vi "Draw Functions.vi"() -> ()   [LabVIEW 2018]
doc: "Draw Functions: This example is an example of drawing functions, demonstrating how to draw lines, rectangles, ellipses, circles, etc."
uses:
  vi.lib/VIRobotics/opencv_yiku/ctls/Size.ctl
  vi.lib/VIRobotics/opencv_yiku/Mat/Create_Mat_8UC3_Size.vi
  vi.lib/VIRobotics/opencv_yiku/opencv_yiku.lvlib
panel:
  in  "pts":cluster{"x":i32, "y":i32}[](array[cluster])
  in  "text":string
  in  "text point":cluster{"x":i32, "y":i32}
  in  "ellipse axes":T1
  in  "ellipse center":cluster{"x":i32, "y":i32}
  in  "circle radius":i32=1
  in  "circle center":cluster{"x":i32, "y":i32}={"x"=200, "y"=200}
  in  "end pt2":cluster{"x":i32, "y":i32}={"x"=350, "y"=270}
  in  "rect":T2={"x"=20, "y"=20, "width"=200, "height"=200}
  in  "end pt":cluster{"x":i32, "y":i32}={"x"=350, "y"=350}
  in  "start pt":cluster{"x":i32, "y":i32}
  out "picture":picture
  # "Overview: Demonstrates how to draw lines, rectangles, ellipses, circles, etc.\nRequirements: Windows.\nInstructions: \n1. Run the VI."
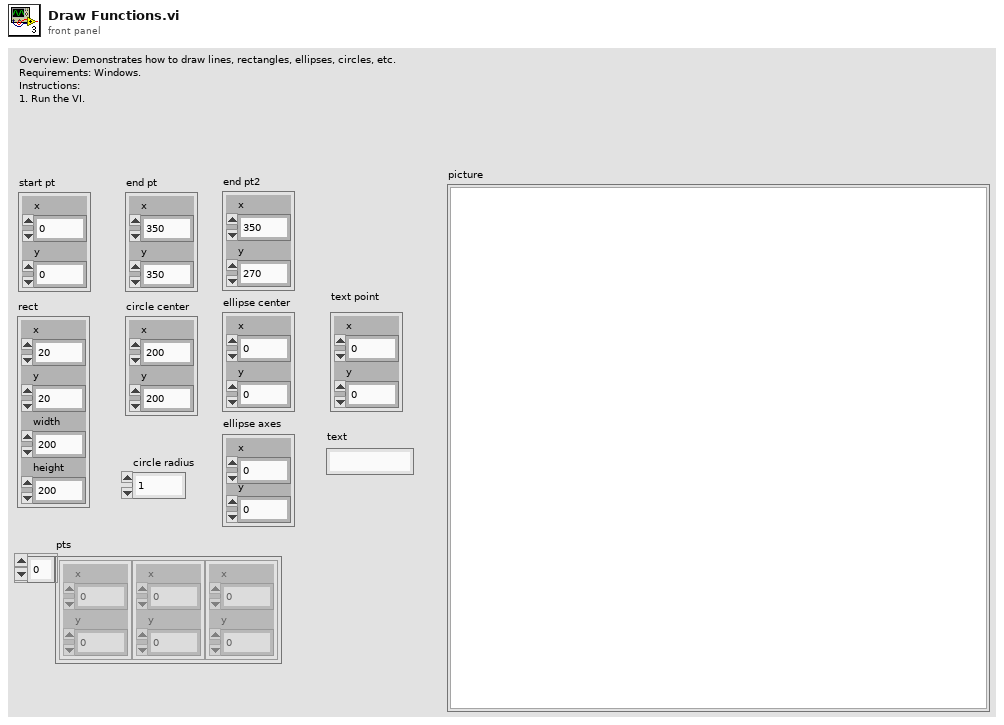
[diagram p1: front panel]
types:
  T1 = typedef "opencv_yiku.lvlib/Size.ctl" = cluster{"x":i32, "y":i32}
  T2 = cluster{"x":i32, "y":i32, "width":i32, "height":i32}
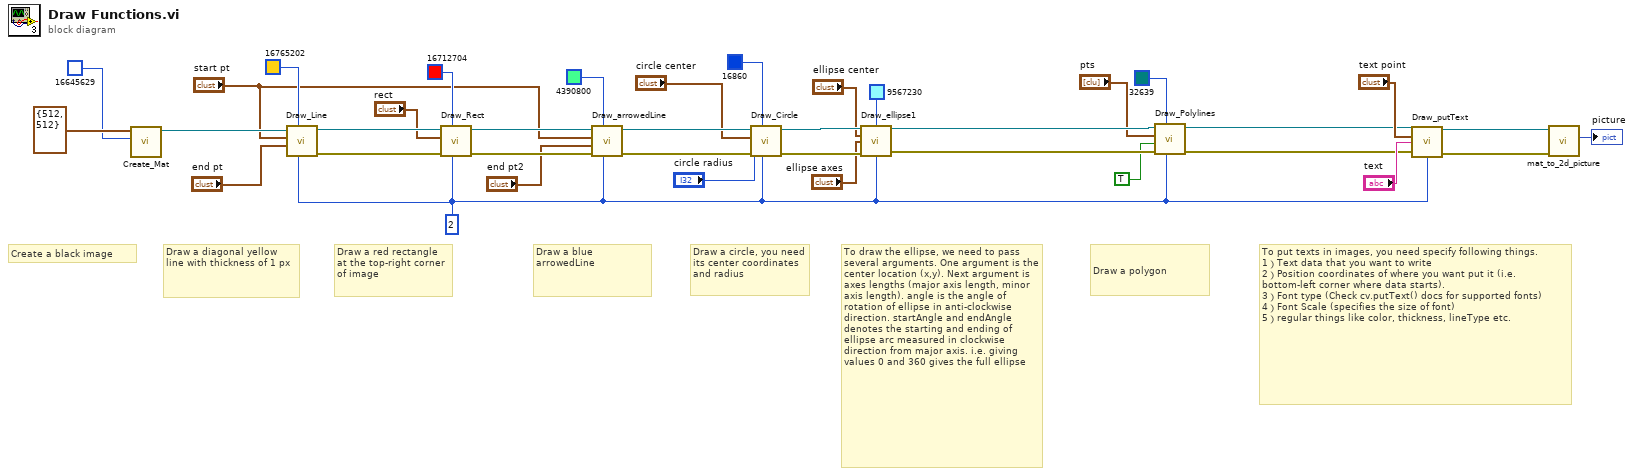
[diagram p0: block diagram]
diagram:
  w5 = 2 ("thickness")
  # "To put texts in images, you need specify following things.\n1）Text data that you want to write\n2）Position coordinates of where you want put it (i.e. bottom-left corner where data starts).\n3）Font type (Check cv.putText() docs for supported fonts)\n4）Font Scale (specifies the size of font)\n5）regular things like color, thickness, lineType etc."
  # "Draw a polygon"
  # "To draw the ellipse, we need to pass several arguments. One argument is the center location (x,y). Next argument is axes lengths (major axis length, minor axis length). angle is the angle of rotation of ellipse in anti-clockwise direction. startAngle and endAngle denotes the starting and ending of ellipse arc measured in clockwise direction from major axis. i.e. giving values 0 and 360 gives the full ellipse"
  # "Draw a circle, you need its center coordinates and radius"
  # "Draw a blue arrowedLine"
  # "Draw a red rectangle at the top-right corner of image"
  # "Draw a diagonal yellow line with thickness of 1 px"
  # "Create a black image"
  n1 = call-poly "Create_Mat.vi"("Color"=u32 16645629, "Size"=cluster{"x":i32, "y":i32} {"x"=512, "y"=512}) -> ("Mat_8U_out"=w34:refnum<class "Mat_8U.lvclass">)  [unwired: 8 in, 1 out]
  n2 = call "Draw_Line.vi"("thickness"=w5, "color"=u32 16765202, "pt2"="end pt", "pt1"="start pt", "Mat"=w34) -> ("error out"=w32:errorcluster, "Mat out"=w33:refnum<class "Mat_8U.lvclass">)  [unwired: 5 in]
  n3 = call "Draw_Rect.vi"("thickness"=w5, "color"=u32 16712704, "error in (no error)"=w32, "rect"="rect", "Mat"=w33) -> ("error out"=w30:errorcluster, "Mat out"=w31:refnum<class "Mat_8U.lvclass">)  [unwired: 5 in]
  n4 = call "Draw_arrowedLine.vi"("thickness"=w5, "color"=u32 4390800, "error in (no error)"=w30, "pt2"="end pt2", "pt1"="start pt", "Mat"=w31) -> ("error out"=w21:errorcluster, "Mat out"=w23:refnum<class "Mat_8U.lvclass">)  [unwired: 4 in]
  n5 = call "Draw_Circle.vi"("thickness"=w5, "color"=u32 16860, "error in (no error)"=w21, "radius"="circle radius", "center"="circle center", "Mat"=w23) -> ("error out"=w17:errorcluster, "Mat out"=w18:refnum<class "Mat_8U.lvclass">)  [unwired: 4 in]
  n6 = call "Draw_ellipse1.vi"("Mat"=w18, "color"=u32 9567230, "center"="ellipse center", "axes"="ellipse axes", "error in (no error)"=w17, "thickness"=w5) -> ("Mat out"=w9:refnum<class "Mat_8U.lvclass">, "error out"=w8:errorcluster)  [unwired: 8 in]
  n7 = call "Draw_Polylines.vi"("thickness"=w5, "color"=u32 32639, "error in (no error)"=w8, "isclosed"=TRUE, "pts"="pts", "Mat"=w9) -> ("error out"=w6:errorcluster, "Mat out"=w7:refnum<class "Mat_8U.lvclass">)  [unwired: 4 in]
  n8 = call "Draw_putText.vi"("Mat"=w7, "point"="text point", "text"="text", "error in (no error)"=w6, "thickness"=w5) -> ("Mat out"=w11:refnum<class "Mat_8U.lvclass">, "error out"=w10:errorcluster)  [unwired: 9 in]
  n9 = call "mat_to_2d_picture.vi"("error in (no error)"=w10, "Mat_8U in"=w11) -> ("picture"=→"picture":picture)  [unwired: 7 in, 2 out]
